vi "Get Circle Grade.vi"(4 "Y":u32=533, 6 "Sin Fixed":fxp<+/-,32,1>[](array[numeric])=[0.0, 0.06342400005087256, 0.126589999999851, 0.18924999982118607, 0.2511499999091029, 0.3120300001464784, 0.37166000017896295, 0.4297899999655783, 0.4862000001594424, 0.5406399997882545, 0.5929100001230836, 0.6427899999544024, 0.6900800000876188, 0.7345900000073016, 0.7761499998159707, 0.8145800000056624, 0.8497299998998642, 0.8814500002190471, 0.9096300001256168, 0.934150000102818, 0.9548999997787178, 0.9718100000172853, 0.984809999819845, 0.9938400001265109, 0.9988699997775257, 0.9998699999414384, 0.9968500002287328, 0.9898199997842312, 0.9788000001572073, 0.9638399998657405, 0.9449999998323619, 0.9223500001244247, 0.8959900001063943, 0.8660300001502037, 0.8325700000859797, 0.7957600001245737, 0.7557500000111759, 0.7126899999566376, 0.6667700000107288, 0.6181600000709295, 0.5670599997974932, 0.513679999858141, 0.45822999998927116, 0.40093000000342727, 0.3420199998654425, 0.2817299999296665, 0.2203099997714162, 0.15799999982118607, 0.09505600016564131, 0.03172799991443753, -0.03172799991443753, -0.09505600016564131, -0.15799999982118607, -0.2203099997714162, -0.2817299999296665, -0.3420199998654425, -0.40093000000342727, -0.45822999998927116, -0.513679999858141, -0.5670599997974932, -0.6181600000709295, -0.6667700000107288, -0.7126899999566376, -0.7557500000111759, -0.7957600001245737, -0.8325700000859797, -0.8660300001502037, -0.8959900001063943, -0.9223500001244247, -0.9449999998323619, -0.9638399998657405, -0.9788000001572073, -0.9898199997842312, -0.9968500002287328, -0.9998699999414384, -0.9988699997775257, -0.9938400001265109, -0.984809999819845, -0.9718100000172853, -0.9548999997787178, -0.934150000102818, -0.9096300001256168, -0.8814500002190471, -0.8497299998998642, -0.8145800000056624, -0.7761499998159707, -0.7345900000073016, -0.6900800000876188, -0.6427899999544024, -0.5929100001230836, -0.5406399997882545, -0.4862000001594424, -0.4297899999655783, -0.37166000017896295, -0.3120300001464784, -0.2511499999091029, -0.18924999982118607, -0.126589999999851, -0.06342400005087256, 0.0], 7 "X":u32=589, 8 "B":u32=334, 9 "Cos Fixed":fxp<+/-,32,1>[](array[numeric])=[0.9999999995343387, 0.9979900000616908, 0.9919500001706183, 0.9819299997761846, 0.967949999962002, 0.9500699997879565, 0.9283699998632073, 0.9029299998655915, 0.8738500000908971, 0.8412500000558794, 0.8052699998952448, 0.7660400001332164, 0.7237300002016127, 0.6785099999979138, 0.6305499998852611, 0.5800600000657141, 0.5272300001233816, 0.472269999794662, 0.4154199999757111, 0.3568899999372661, 0.29692000010982156, 0.23576000006869435, 0.17364999977871776, 0.11084000021219254, 0.04758200002834201, -0.015866000205278397, -0.07924999995157123, -0.14231000002473593, -0.20481000002473593, -0.2664700001478195, -0.327070000115782, -0.3863499998115003, -0.4440700002014637, -0.5, -0.5539199998602271, -0.6056099999696016, -0.6548600001260638, -0.7014700002036989, -0.7452600002288818, -0.7860500002279878, -0.8236799999140203, -0.8579799998551607, -0.8888400001451373, -0.9161100001074374, -0.9396899999119341, -0.9594899998046458, -0.9754300001077354, -0.9874399998225272, -0.9954699999652803, -0.9994999999180436, -0.9994999999180436, -0.9954699999652803, -0.9874399998225272, -0.9754300001077354, -0.9594899998046458, -0.9396899999119341, -0.9161100001074374, -0.8888400001451373, -0.8579799998551607, -0.8236799999140203, -0.7860500002279878, -0.7452600002288818, -0.7014700002036989, -0.6548600001260638, -0.6056099999696016, -0.5539199998602271, -0.5, -0.4440700002014637, -0.3863499998115003, -0.327070000115782, -0.2664700001478195, -0.20481000002473593, -0.14231000002473593, -0.07924999995157123, -0.015866000205278397, 0.04758200002834201, 0.11084000021219254, 0.17364999977871776, 0.23576000006869435, 0.29692000010982156, 0.3568899999372661, 0.4154199999757111, 0.472269999794662, 0.5272300001233816, 0.5800600000657141, 0.6305499998852611, 0.6785099999979138, 0.7237300002016127, 0.7660400001332164, 0.8052699998952448, 0.8412500000558794, 0.8738500000908971, 0.9029299998655915, 0.9283699998632073, 0.9500699997879565, 0.967949999962002, 0.9819299997761846, 0.9919500001706183, 0.9979900000616908, 0.9999999995343387], 10 "Picture":u8[][](array[numeric]), 11 "A":u32=337) -> (3 "Grade":u32)   [LabVIEW 2015]
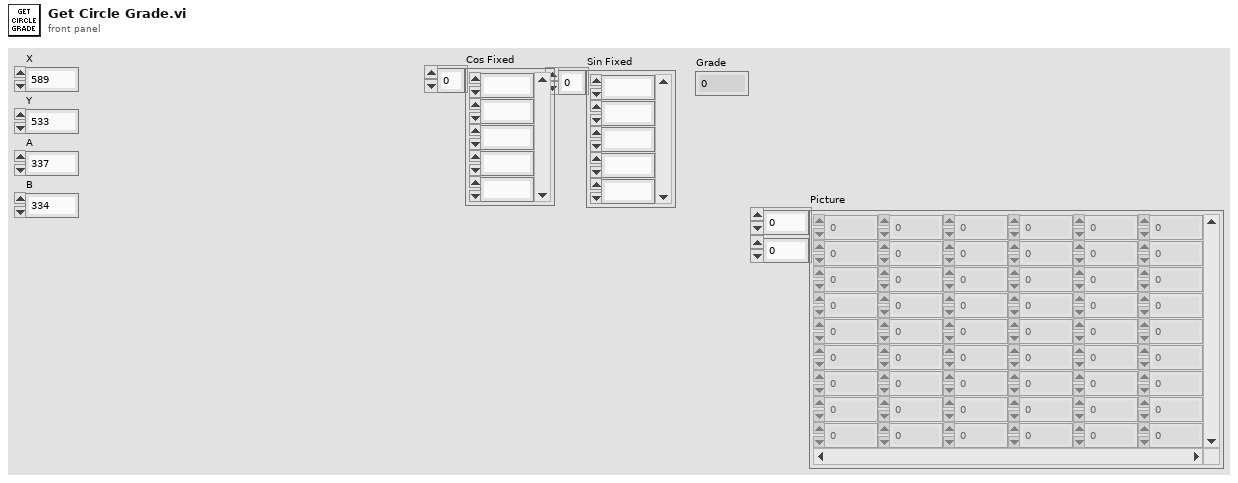
[diagram p1: front panel]
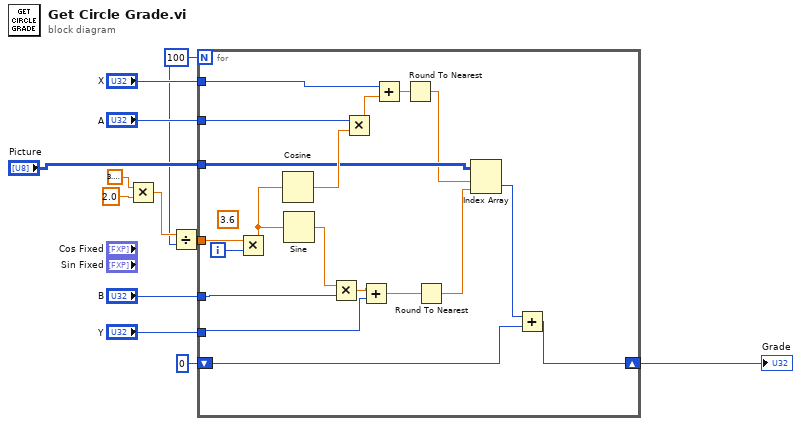
[diagram p0: block diagram]
diagram:
  w2 = 100
  n1 = Multiply(x=3.141592653589793, y=2.0) -> (x*y=w3:dbl)
  n2 = Divide(x=w3, y=w2) -> (x/y=w1:dbl)
  n3 = for {
    N: w2 -> [_]
    tunnel: "A" -> [w28]
    tunnel: "X" -> [w26]
    tunnel: "Y" -> [w22]
    shift-right: [w29] -> w12
    shift-left: u32 0 -> [w30]
    tunnel: "B" -> [w24]
    tunnel: w1 -> [w16]
    tunnel: "Picture" -> [w15]
    i -> [w20]
    (unwired) 3.6
    n4 = Multiply(x=w16, y=w20) -> (x*y=w19:dbl)
    n5 = Cosine(x=w19) -> (cos(x)=w17:dbl)
    n6 = Sine(x=w19) -> (sin(x)=w18:dbl)
    n7 = Multiply(x=w18, y=w24) -> (x*y=w23:dbl)
    n8 = Multiply(x=w28, y=w17) -> (x*y=w27:dbl)
    n9 = Add(x=w23, y=w22) -> (x+y=w21:dbl)
    n10 = Add(x=w26, y=w27) -> (x+y=w25:dbl)
    n11 = Round To Nearest(number=w25) -> (nearest integer value=w14:dbl)
    n12 = Round To Nearest(number=w21) -> (nearest integer value=w13:dbl)
    n13 = Index Array(array=w15, index (row)=w14, index (col)=w13) -> (element=w31:u8)
    n14 = Add(x=w31, y=w30) -> (x+y=w29:u32)
  }
  "Grade" <- w12
